vi "845x_SPI Read.vi"(0 "Device":T1, 1 "I/O Voltage Level":i32(ring)=33 items=["3.3V"=33, "2.5V"=25, "1.8V"=18, "1.5V"=15, "1.2V"=12], 5 "Chip Select":u32, 7 "Clock Rate (kHz)":u16=1000, 9 "EEPROM Data Address":u16 format="%.0x", 11 "error in (no error)":errorcluster, 12 "Number of Bytes to Read":i32=32 max=8192 step=1, 13 "Data Address Width":enum16{"1 Byte", "2 Byte"}(ring)=enum."2 Byte", 14 "Data Address Endianness":bool=TRUE) -> (4 "Read Data":u8[](array[numeric]) format="%x", 15 "error out":errorcluster)   [LabVIEW 2021, in "Communication.lvlib"]
doc: "<B>NOTE: This example is taken from ni845x driver examples located at C:\\Program Files (x86)\\National Instruments\\LabVIEW <version>\\examples\\ni845x\\845xEx.llb. More such examples can be found in the same location.</B>\n\nThis example shows a more generalized way to use the SPI basic API to read data. It allows the user to change the following parameters: the endianness of the address bytes, and the number of bytes in an address.\n\nThe parameters will have the following effects:\n\nData Address Width: This will allow the user to specify the EEPROM Data Address as either 1 or 2 bytes.\nData Address Endianness: This control will change the ordering of the bytes in the EEPROM Data Address, note that this only has an effect if there are 2 bytes in the address.\n\nFor connection information see the NI-845x Hardware and Software manual and the manual for your specific SPI device."
uses:
  Communication.lvlib
  <vilib>/ni845x/ni845x.llb/ni845xControl.ctl
  <vilib>/ni845x/ni845x.llb/NI-845x SPI Close Configuration Reference.vi
  <resource>/objmgr/NI845x.rc
panel:
  # "See VI Info <Ctrl+I> for more information on how to use this example"
  # "Device Configuration"
  # "SPI Data"
  # "SPI Slave Configuration"
  # "Big Endian"
  # "Little Endian"
  # "NOTE: This example is taken from ni845x driver examples located at C:\\Program Files (x86)\\National Instruments\\LabVIEW <version>\\examples\\ni845x\\845xEx.llb.  More such examples can be found in the same location."
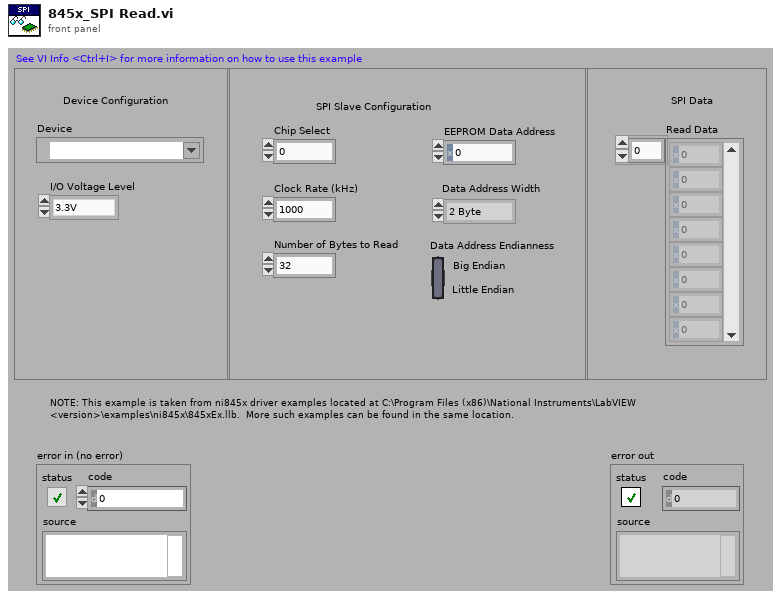
[diagram p1: front panel]
types:
  T1 = typedef "ni845xControl.ctl" = refnum<k21>
  T2 = typedef "ni845xSpiConfiguration.ctl" = refnum<k20>
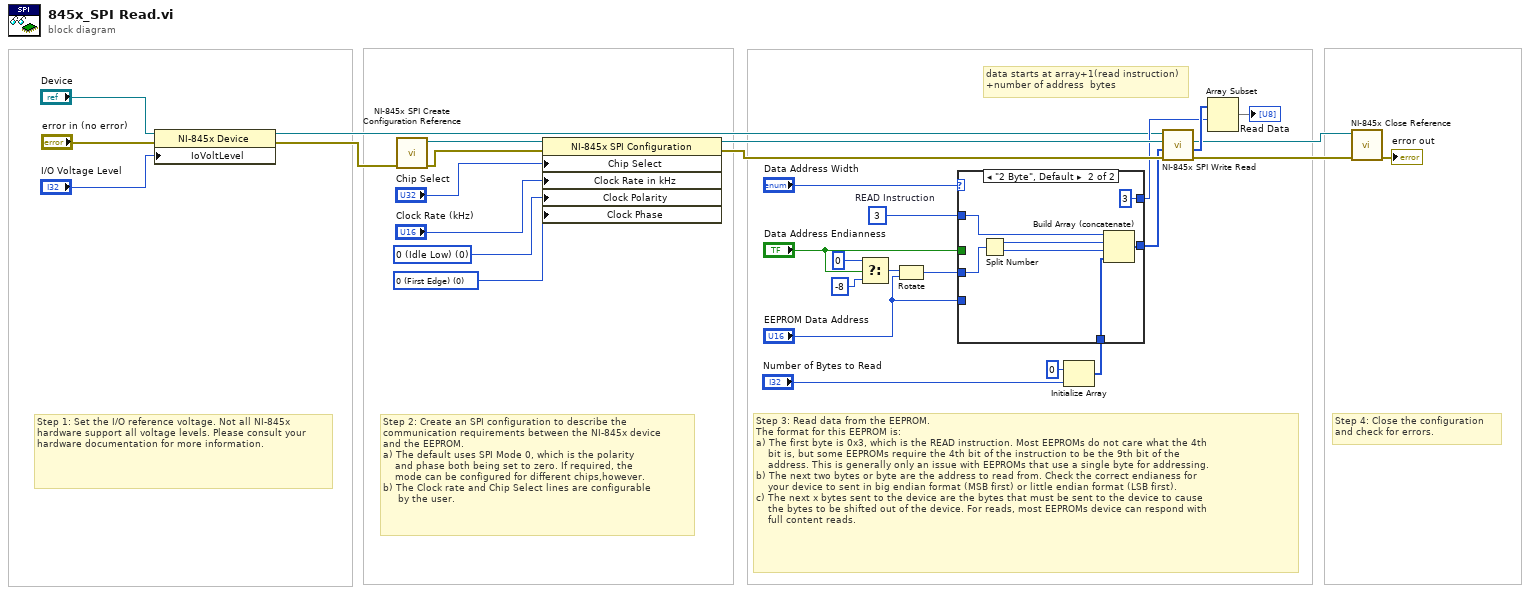
[diagram p0: block diagram]
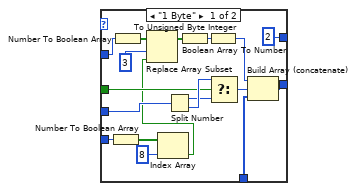
[diagram p2: hidden frame]
diagram:
  w30 = 0 items=["0 (First Edge)", "1 (Second Edge)"] ("Clock Phase")
  w31 = 0 items=["0 (Idle Low)", "1 (Idle High)"] ("Clock Polarity")
  w18 = u8 3  # READ Instruction
  # "Step 1: Set the I/O reference voltage. Not all NI-845x hardware support all voltage levels. Please consult your hardware documentation for more information."
  # "Step 4: Close the configuration \nand check for errors."
  # "data starts at array+1(read instruction)\n+number of address  bytes"
  # "Step 2: Create an SPI configuration to describe the \ncommunication requirements between the NI-845x device \nand the EEPROM.\na) The default uses SPI Mode 0, which is the polarity \n    and phase both being set to zero. If required, the\n    mode can be configured for different chips,however. \nb) The Clock rate and Chip Select lines are configurable \n     by the user."
  # "Step 3: Read data from the EEPROM. \nThe format for this EEPROM is:\na) The first byte is 0x3, which is the READ instruction. Most EEPROMs do not care what the 4th \n    bit is, but some EEPROMs require the 4th bit of the instruction to be the 9th bit of the \n    address. This is generally only an issue with EEPROMs that use a single byte for addressing.\nb) The next two bytes or byte are the address to read from. Check the correct endianess for \n    your device to sent in big endian format (MSB first) or little endian format (LSB first).\nc) The next x bytes sent to the device are the bytes that must be sent to the device to cause \n    the bytes to be shifted out of the device. For reads, most EEPROMs device can respond with \n    full content reads."
  n1 = property on="Property Node" class="NI-845x Device"(reference="Device", error in="error in (no error)", "IoVoltLevel"="I/O Voltage Level") -> (reference out=w4:T1, error out=w3:errorcluster)
  n2 = call <vilib>:"NI-845x SPI Create Configuration Reference.vi"("error in (no error)"=w3) -> ("error out"=w21:errorcluster, "spi configuration"=w22:T2)  [unwired: 9 out]
  n3 = property class="NI-845x SPI Configuration"(reference=w22, error in=w21, "Chip Select"="Chip Select", "Clock Rate in kHz"="Clock Rate (kHz)", "Clock Polarity"=w31, "Clock Phase"=w30) -> (reference out=w27:T2, error out=w26:errorcluster)
  n4 = Select(t=i16 0, s="Data Address Endianness", f=i16 -8) -> (s? t:f=w13:i16)
  n5 = Rotate(1:"EEPROM Data Address", 2:w13) -> (0:w12:u16)
  n6 = Initialize Array(u8 0 ("element"), "Number of Bytes to Read") -> (w9:u8[])
  n7 = case shown="\"2 Byte\", Default" "Data Address Width" {
    tunnel: w18 -> [w38 w53]
    tunnel: [w49 w54] -> w10
    tunnel: [2 ("index") 3 ("index")] -> w14
    tunnel: w12 -> [w47 w51]
    tunnel: "Data Address Endianness" -> [w43 _]
    tunnel: w9 -> [w36 w50]
    tunnel: "EEPROM Data Address" -> [w32 _]
    frame "1 Byte" {
      n8 = Number To Boolean Array(number=w32) -> (Boolean array=w34:bool[])
      n9 = Number To Boolean Array(number=w38) -> (Boolean array=w40:bool[])
      n10 = Index Array(array=w34, index=8) -> (element=w33:bool)
      n11 = Replace Array Subset(array=w40, new element=w33, index=3) -> (w41:bool[])
      n12 = Split Number(x=w47) -> (hi(x)=w45:u8, lo(x)=w46:u8)
      n13 = Boolean Array To Number(Boolean array=w41) -> (number=w42:u32)
      n14 = To Unsigned Byte Integer(number=w42) -> (unsigned 8bit integer=w37:u8)
      n15 = Select(t=w46, s=w43, f=w45) -> (s? t:f=w44:u8)
      n16 = Build Array (concatenate)(w37, w44, w36) -> (w49:u8[])
    }
    frame "2 Byte", Default {
      n17 = Split Number(x=w51) -> (hi(x)=w56:u8, lo(x)=w55:u8)
      n18 = Build Array (concatenate)(w53, w56, w55, w50) -> (w54:u8[])
    }
  }
  n19 = call <vilib>:"NI-845x SPI Write Read.vi"("error in (no error)"=w26, "write data"=w10, "spi configuration in"=w27, "device reference in"=w4) -> ("error out"=w20:errorcluster, "read data"=w23:u8[], "spi configuration out"=w19:T2)  [unwired: 5 out]
  n20 = Array Subset(array=w23, index=w14) -> (→"Read Data":u8[])  [unwired: 1 in]
  n21 = call-poly <vilib>:"NI-845x Close Reference.vi"("error in (no error)"=w20, "spi configuration"=w19) -> ("error out"=→"error out":errorcluster)  [unwired: 9 out]
